vi "can port ui.vi"() -> ()   [LabVIEW 2013, in "can port.lvclass"]
uses:
  can port.lvclass
  <vilib>/NI/Configuration Framework/Node/NodeRef.ctl
  <vilib>/NI/Configuration Framework/Node/NISE_CEF_Node.lvclass
  <vilib>/NI/AMC/Message Queue.ctl
  <vilib>/NI/AMC/Message.ctl
  <vilib>/NI/Tools/Keyed Array/KeyedArray.ctl
  <vilib>/NI/Configuration Framework/Node/UserEventRef.ctl
  <vilib>/NI/Configuration Framework/Controls/EventCluster.ctl
  can port.lvclass/can port.ctl
  <vilib>/NI/Tools/Keyed Array/Tools_KeyedArray.lvlib
  <vilib>/NI/AMC/AMC.lvlib
  <vilib>/NI/Configuration Framework/NISE_CEF_TreeControl.lvlib
panel:
  in  "Name":u64
  in  "J1939 Network Address":u8
  in  "BaudRate":u32
  in  "user event":T1
  in  "main queue":T2
  in  "node ref":T3
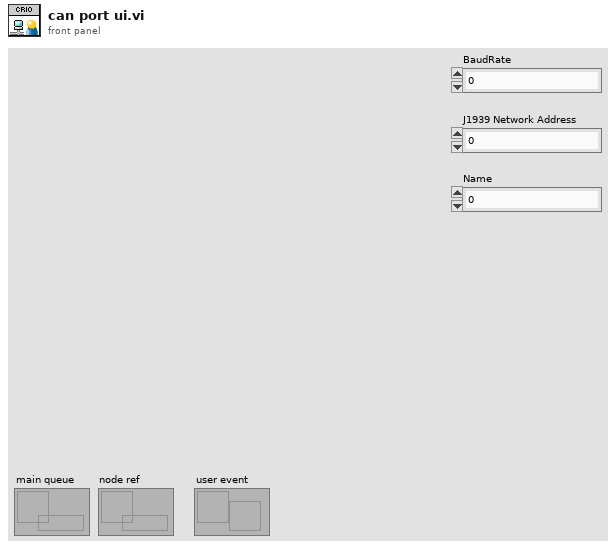
[diagram p1: front panel]
types:
  T1 = typedef "NISE_CEF_Node.lvclass/UserEventRef.ctl" = refnum<user-event>
  T2 = typedef "AMC.lvlib/Message Queue.ctl" = refnum<queue>
  T3 = typedef "NISE_CEF_Node.lvclass/NodeRef.ctl" = refnum<data-value>
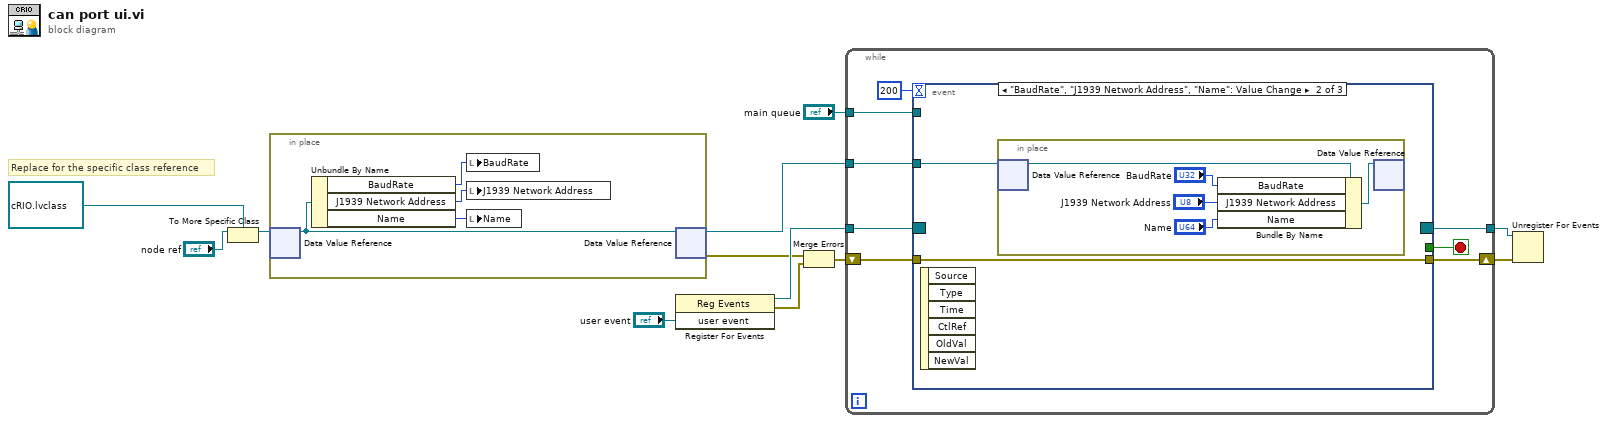
[diagram p0: block diagram]
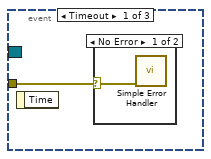
[diagram p2: hidden frame]
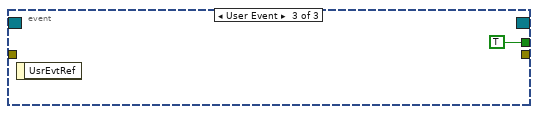
[diagram p4: hidden frame]
diagram:
  # "Replace for the specific class reference"
  n1 = To More Specific Class(target class=refnum<data-value> refnum ("data value reference"), reference="node ref") -> (specific class reference=w5:refnum<data-value>)  [unwired: 1 in, 1 out]
  n2 = in-place {
    n3 = in-place-dvr #1(w5) -> (w16:refnum<class "can port.lvclass">)  [unwired: 1 out]
    n4 = Unbundle By Name(w16) -> ("BaudRate"=w15:u32, "J1939 Network Address"=w13:u8, "Name"=w14:u64)
    n5 = local write "BaudRate"(w15) -> ()
    n6 = local write "J1939 Network Address"(w13) -> ()
    n7 = local write "Name"(w14) -> ()
    n8 = in-place-dvr #1(w16) -> (w12:refnum<data-value>, w2:errorcluster)
  }
  n9 = register-events("user event") -> (reference out=w9:refnum<event-registration>, error out=w3:errorcluster)  [unwired: 2 in]
  n10 = Merge Errors(w2, w3) -> (w1:errorcluster)
  n11 = while {
    tunnel: w12 -> [w24]
    tunnel: "main queue" -> [w23]
    tunnel: w9 -> [w21]
    tunnel: [w20] -> w8
    shift-right: [w18] -> w7
    shift-left: w1 -> [w17]
    stop <- w19 stop-if-true
    n12 = event shown="[1] \"BaudRate\", \"J1939 Network Address\", \"Name\": Value Change" {
      selector: w21 -> [_ _ _]
      dyn-events: [_ _ _] -> w20
      timeout: 200 -> [_ _ _]
      tunnel: w24 -> [_ w28 _]
      tunnel: w23 -> [_ _ _]
      tunnel: [_ _ TRUE] -> w19
      tunnel: [_ w27 _] -> w18
      tunnel: w17 -> [w25 w27 _]
      event Timeout {
        n13 = event-data() -> ()  [unwired: 1 in, 1 out]
        n14 = case shown="No Error" w25 {
          selector: w25 -> [w26 _]
          frame No Error {
            n15 = call <vilib>:"Simple Error Handler.vi"("error in (no error)"=w26) -> ()  [unwired: 4 in, 5 out]
          }
          frame Error {
          }
        }
      }
      event "BaudRate", "J1939 Network Address", "Name": Value Change {
        n16 = event-data() -> ()  [unwired: 1 in, 6 out]
        n17 = in-place {
          n18 = in-place-dvr #2(w28) -> (w33:refnum<class "can port.lvclass">)  [unwired: 1 out]
          n19 = Bundle By Name(cluster=w33, "BaudRate"="BaudRate", "J1939 Network Address"="J1939 Network Address", "Name"="Name") -> (w32:refnum<class "can port.lvclass">)
          n20 = in-place-dvr #2(w32) -> ()  [unwired: 2 out]
        }
      }
      event User Event {
        n21 = event-data() -> ()  [unwired: 1 in, 1 out]
      }
    }
  }
  n22 = Unregister For Events(event registration refnum=w8, error in=w7) -> ()  [unwired: 1 out]
